vi "Write RepRate.vi"(8 "error in (no error)":errorcluster, 10 "RepRate":u16, 11 "Change Laser Rep Rate CMD in":refnum<class "Change Laser Rep Rate CMD.lvclass">) -> (0 "error out":errorcluster, 3 "Change Laser Rep Rate CMD out":refnum<class "Change Laser Rep Rate CMD.lvclass">)   [LabVIEW 2016, in "gCRDS.lvlib" / "Change Laser Rep Rate CMD.lvclass"]
uses:
  Change Laser Rep Rate CMD.lvclass
  Change Laser Rep Rate CMD.lvclass/Change Laser Rep Rate CMD.ctl
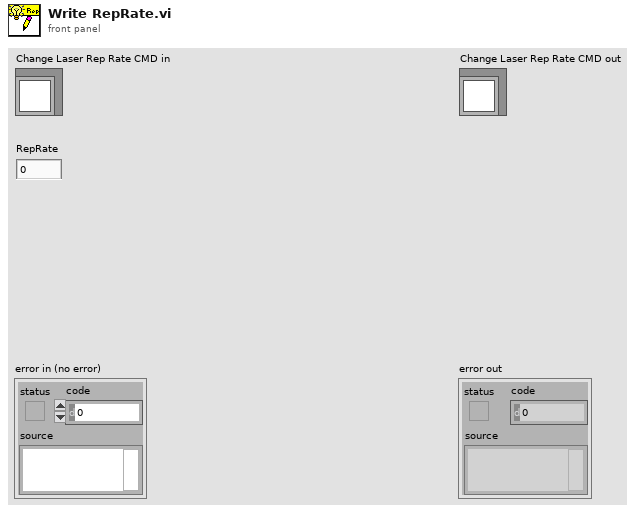
[diagram p1: front panel]
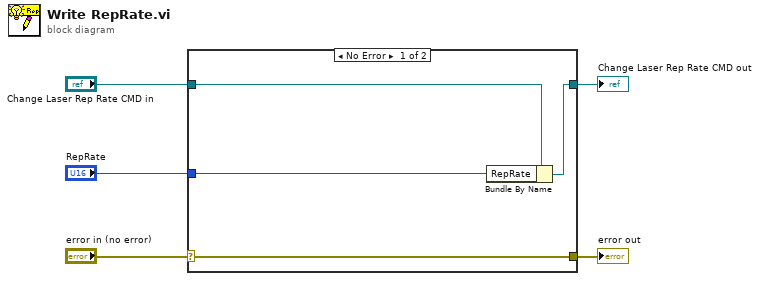
[diagram p0: block diagram]
diagram:
  n1 = case shown="No Error" "error in (no error)" {
    selector: "error in (no error)" -> [w9 w10]
    tunnel: [w9 w10] -> w4
    tunnel: [w7 w11] -> w2
    tunnel: "Change Laser Rep Rate CMD in" -> [w8 w11]
    tunnel: "RepRate" -> [w6 _]
    frame No Error {
      n2 = Bundle By Name(cluster=w8, "RepRate"=w6) -> (w7:refnum<class "Change Laser Rep Rate CMD.lvclass">)
    }
    frame Error {
    }
  }
  "error out" <- w4
  "Change Laser Rep Rate CMD out" <- w2
